vi "svacg_FrequencyResponse Convert Phase.vi"(7 "Response delay (s)":dbl, 9 "Ignore timestamp":bool=TRUE, 10 "View":T1={"Mag. in dB"=TRUE, "Unwrap phase"=FALSE, "Phase in deg."=TRUE}, 11 "phase (radians) in":cluster{"f0":dbl, "df":dbl, "phase":dbl[]} {"phase" format="%.2p"; "f0" format="%0.2p"; "df" format="%0.2p"}) -> (2 "phase unit label":string="deg", 3 "converted phase out":cluster{"f0":dbl, "df":dbl, "phase":dbl[]} {"phase" format="%.2p"; "f0" format="%0.2p"; "df" format="%0.2p"})   [LabVIEW 2017]
uses:
  <vilib>/Analysis/NI_AALPro.lvlib
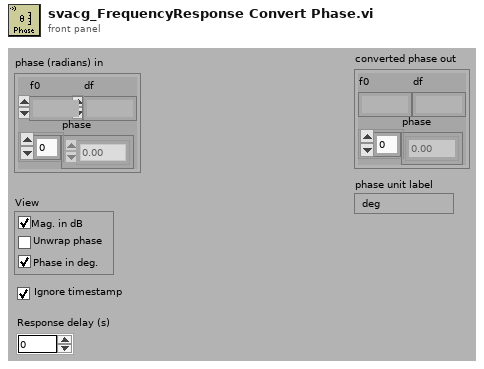
[diagram p1: front panel]
types:
  T1 = cluster{"Mag. in dB":bool, "Unwrap phase":bool, "Phase in deg.":bool}
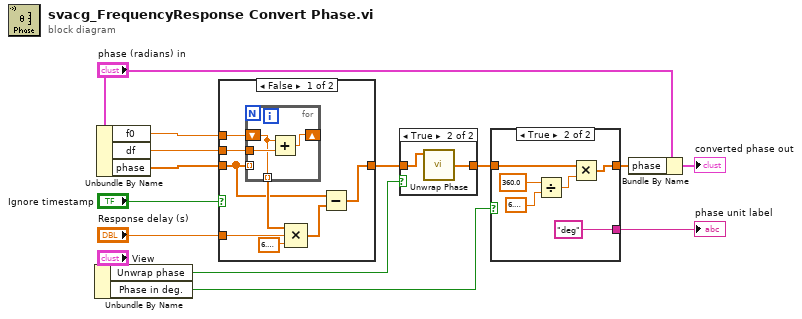
[diagram p0: block diagram]
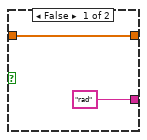
[diagram p4: hidden frame]
diagram:
  n1 = Unbundle By Name("View") -> ("Unwrap phase"=w8:bool, "Phase in deg."=w9:bool)
  n2 = Unbundle By Name("phase (radians) in") -> ("f0"=w4:dbl, "df"=w3:dbl, "phase"=w5:dbl[])
  n3 = case shown="False" "Ignore timestamp" {
    tunnel: [w15 w26] -> w6
    tunnel: w5 -> [w17 w26]
    tunnel: w4 -> [w22 _]
    tunnel: w3 -> [w21 _]
    tunnel: "Response delay (s)" -> [w19 _]
    frame False {
      n4 = for {
        tunnel: w17 -> [_] mode=indexing
        shift-right: [w25] -> _
        shift-left: w22 -> [w23]
        tunnel: w21 -> [w24]
        tunnel: [w23] -> w20 mode=indexing
        n5 = Add(x=w23, y=w24) -> (x+y=w25:dbl)
      }
      n6 = Compound Arithmetic op=MULTIPLY(w20, w19, 6.283185307179586) -> (w16:dbl[])
      n7 = Subtract(x=w17, y=w16) -> (x-y=w15:dbl[])
    }
    frame True {
    }
  }
  n8 = case shown="True" w8 {
    tunnel: w6 -> [w27 w29]
    tunnel: [w27 w28] -> w14
    frame False {
    }
    frame True {
      n9 = call <vilib>:"Unwrap Phase.vi"("Phase"=w29) -> ("Unwrapped Phase"=w28:dbl[])  [unwired: 9 in, 1 out]
    }
  }
  n10 = case shown="True" w9 {
    tunnel: [w31 w36] -> w12
    tunnel: w14 -> [w31 w37]
    tunnel: ["rad" "deg"] -> w1
    frame False {
    }
    frame True {
      n11 = Divide(x=360.0, y=6.283185307179586) -> (x/y=w33:dbl)
      n12 = Multiply(x=w37, y=w33) -> (x*y=w36:dbl[])
    }
  }
  "phase unit label" <- w1
  n13 = Bundle By Name(cluster="phase (radians) in", "phase"=w12) -> (→"converted phase out":cluster{"f0":dbl, "df":dbl, "phase":dbl[]})
